vi "Calibrate pump waveplate.vi"(0 "VISA Refnum in":refnum<visa-resource-name>, 1 "Trigger rate \nat maximum":dbl, 2 "Mode":enum16{"Constant power", "Constant time"}(ring), 3 "Trigger rate warnings?":bool, 5 "Target trial \nlength (ms)":dbl, 7 "Target trigger rate":dbl, 8 "Threshold":dbl, 9 "Photon #":i32, 11 "error in (no error)":errorcluster, 13 "N":i32=5, 14 "Axis in":i32=3) -> (4 "VISA Refnum out":refnum<visa-resource-name>, 6 "WP position":dbl, 10 "WP Error":bool=TRUE, 15 "error out":errorcluster)   [LabVIEW 2013]
uses:
  <vilib>/imath/engines/lvmath2/RunTimeEngine/BuiltInFunctions/asin/NIMS_asin(C).vi
  <instcachedir>/0/NIMS_asin(C)_73B68F6B04904A8785972686F67E90FD.lvgen/NIMS_asin(C)_73B68F6B04904A8785972686F67E90FD_001.vi
  <vilib>/imath/engines/lvmath2/RunTimeEngine/NodeEndStatement/NIMS_NodeEndStatement_Output.vi
  <instcachedir>/0/NIMS_NodeEndStatement_Output_53EC0D466D134D7ABD903AC30B43404B.lvgen/NIMS_NodeEndStatement_Output_53EC0D466D134D7ABD903AC30B43404B_010.vi
  <instcachedir>/0/NIMS_NodeEndStatement_Output_53EC0D466D134D7ABD903AC30B43404B.lvgen/NIMS_NodeEndStatement_Output_53EC0D466D134D7ABD903AC30B43404B_001.vi
  <vilib>/imath/engines/lvmath2/RunTimeEngine/BuiltInFunctions/abs/NIMS_abs(signed).vi
  <instcachedir>/0/NIMS_abs(signed)_C4FCB8E6058B49B797C7C8D53CA5F6EC.lvgen/NIMS_abs(signed)_C4FCB8E6058B49B797C7C8D53CA5F6EC_000.vi
  <vilib>/imath/engines/lvmath2/RunTimeEngine/ErrorHandling/NIMS_Finalize Error.vi
  <instcachedir>/0/NIMS_NodeEndStatement_Output_53EC0D466D134D7ABD903AC30B43404B.lvgen/NIMS_NodeEndStatement_Output_53EC0D466D134D7ABD903AC30B43404B_009.vi
  <instcachedir>/0/NIMS_abs(signed)_C4FCB8E6058B49B797C7C8D53CA5F6EC.lvgen/NIMS_abs(signed)_C4FCB8E6058B49B797C7C8D53CA5F6EC_002.vi
panel:
  out "t_ratio":dbl
  out "Time":dbl
  out "Calculated trial length":dbl
  out "theta1":dbl
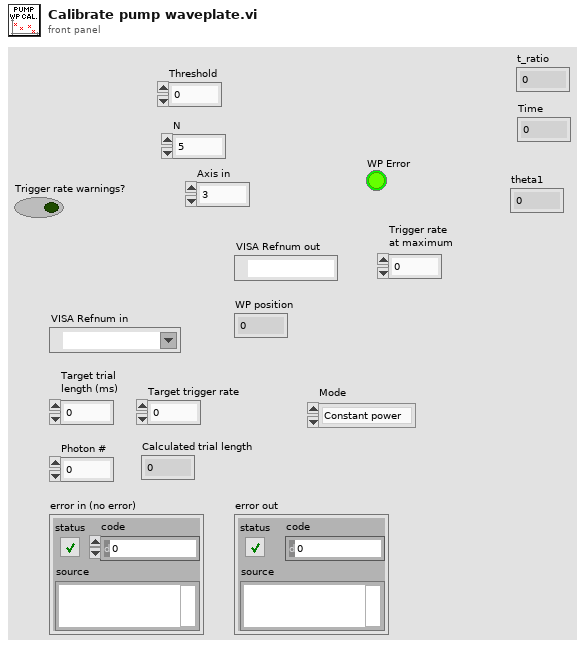
[diagram p1: front panel]
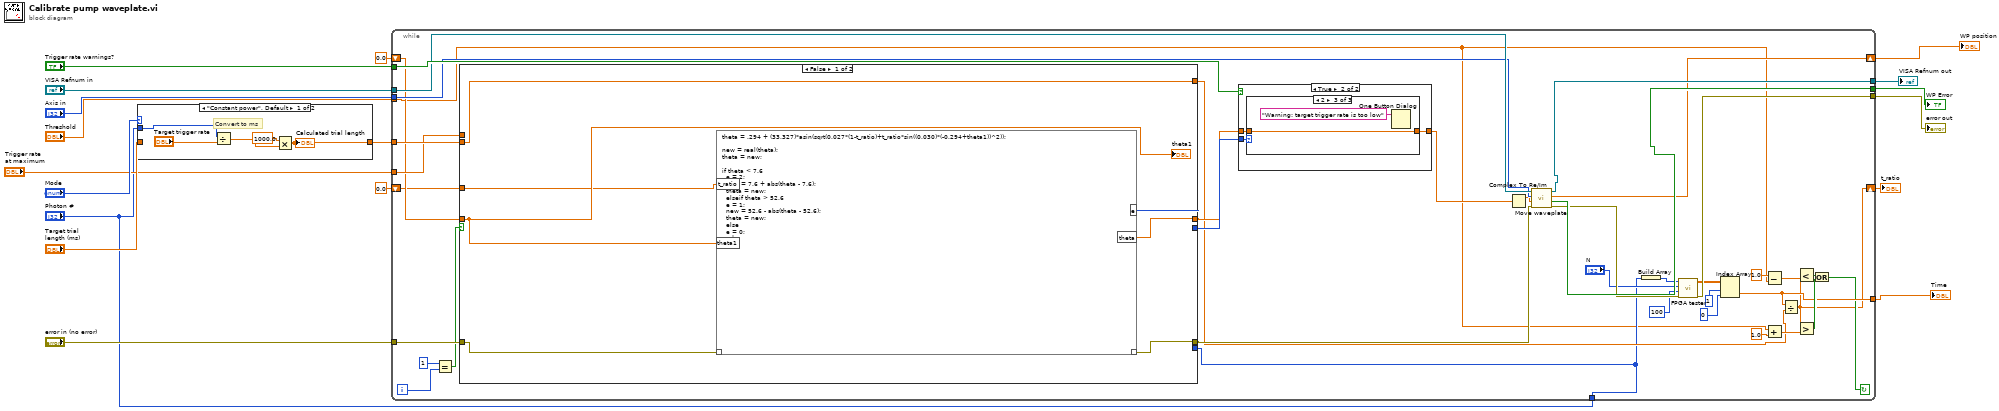
[diagram p0: block diagram]
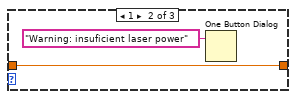
[diagram p4: hidden frame]
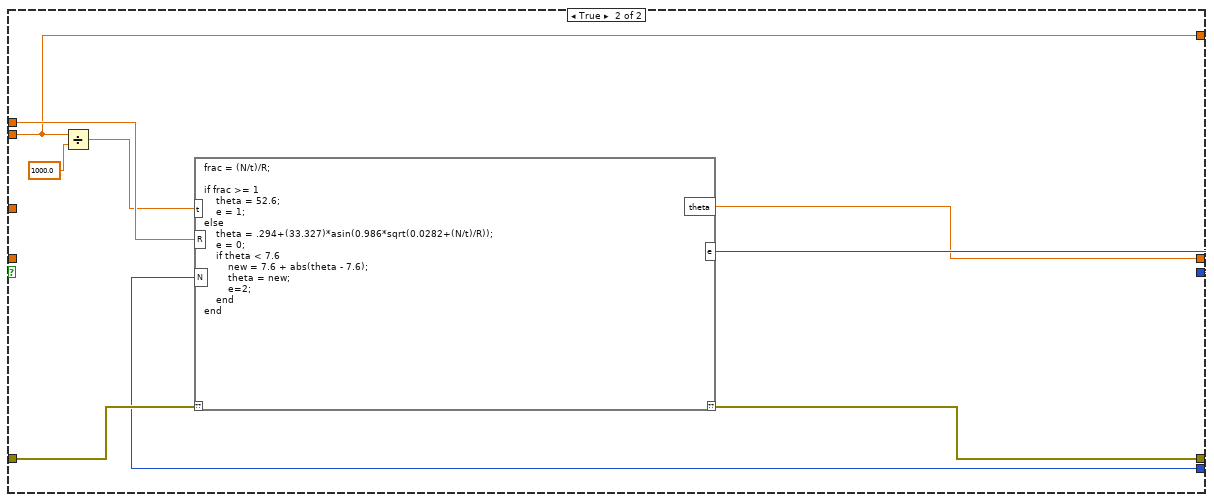
[diagram p5: hidden frame]
diagram:
  n1 = case shown="\"Constant power\", Default" "Mode" {
    tunnel: [w19 w24] -> w12
    tunnel: "Target trial \nlength (ms)" -> [_ w24]
    tunnel: "Photon #" -> [w23 _]
    frame "Constant power", Default {
      # "Convert to ms"
      n2 = Divide(x=w23, y="Target trigger rate") -> (x/y=w21:dbl)
      n3 = Multiply(x=1000.0, y=w21) -> (x*y=w19:dbl)
      "Calculated trial length" <- w19
    }
    frame "Constant time" {
    }
  }
  n4 = while {
    tunnel: "error in (no error)" -> [w63]
    tunnel: "Trigger rate warnings?" -> [w62]
    tunnel: [w61] -> w16
    tunnel: [w60] -> w15
    tunnel: [w45] -> w13
    tunnel: w12 -> [w59]
    tunnel: "Threshold" -> [w25]
    tunnel: "VISA Refnum in" -> [w49]
    tunnel: "Axis in" -> [w48]
    tunnel: "Trigger rate \nat maximum" -> [w58]
    tunnel: "Photon #" -> [w26]
    shift-right: [w50] -> w14
    shift-left: 0.0 ("Current position (units)") -> [w39]
    shift-right: [w29] -> w1
    shift-left: 0.0 -> [w28]
    tunnel: [w32] -> w4
    i -> [w53]
    stop <- w30 continue-if-true
    n5 = Equal?(x=1, y=w53) -> (x = y?=w52:bool)
    n6 = case shown="False" w52 {
      tunnel: w58 -> [_ w215]
      tunnel: [w76 w209] -> w56
      tunnel: [w79 w214] -> w57
      tunnel: w59 -> [w74 w207]
      tunnel: w63 -> [w78 w213]
      tunnel: [w77 w212] -> w51
      tunnel: w39 -> [w75 _]
      tunnel: [w74 w207] -> w31
      tunnel: w28 -> [w73 _]
      tunnel: w26 -> [_ w208]
      frame False {
        n7 = mathscript code="theta = .294 + (33.327)*asin(sqrt(0.027*(1-t_ratio)+t_ratio*sin((0.030)*(-0.294+theta1))^2));\n\nnew = real(theta);\ntheta = new;\n\nif theta < 7.6\n  e = 2;\n  new = 7.6 + abs(theta - 7.6);\n  theta = new;\n  elseif theta > 52.6\n  e = 1;\n  new = 52.6 - abs(theta - 52.6);\n  theta = new;\n  else\n  e = 0;\nend"("??"=w78, "t_ratio"=w73, "theta1"=w75) -> ("??"=w77:errorcluster, "e"=w79:i32, "theta"=w76:dbl)
        "theta1" <- w75
      }
      frame True {
        n8 = Divide(x=w207, y=1000.0) -> (x/y=w210:dbl)
        n9 = mathscript code="frac = (N/t)/R;\n\nif frac >= 1\n    theta = 52.6;\n    e = 1;\nelse\n    theta = .294+(33.327)*asin(0.986*sqrt(0.0282+(N/t)/R));\n    e = 0;\n    if theta < 7.6\n        new = 7.6 + abs(theta - 7.6);\n        theta = new;\n        e=2;\n    end\nend"("??"=w213, "t"=w210, "R"=w215, "N"=w208) -> ("??"=w212:errorcluster, "e"=w214:i32, "theta"=w209:cdb)
      }
    }
    n10 = case shown="True" w62 {
      tunnel: [w64 w67] -> w55
      tunnel: w56 -> [w64 w66]
      tunnel: w57 -> [_ w65]
      frame False {
      }
      frame True {
        n11 = case shown="2" w65 {
          tunnel: w66 -> [w68 w69 w71]
          tunnel: [w68 w69 w71] -> w67
          frame 0, Default {
          }
          frame 1 {
            n12 = One Button Dialog(message="Warning: insuficient laser power") -> ()  [unwired: 1 in, 1 out]
          }
          frame 2 {
            n13 = One Button Dialog(message="Warning: target trigger rate is too low") -> ()  [unwired: 1 in, 1 out]
          }
        }
      }
    }
    n14 = Complex To Re/Im(x + iy=w55) -> (x=w47:dbl)  [unwired: 1 out]
    n15 = call "Move waveplate.vi"("error in (no error)"=w51, "Angle"=w47, "Axis in"=w48, "VISA Refnum in"=w49) -> ("error out"=w46:errorcluster, "WP Error"=w60:bool, "Current position (units)"=w50:dbl, "VISA Refnum out"=w61:refnum<visa-resource-name>)  [unwired: 4 in]
    n16 = Build Array(w26) -> (w44:i32[])
    n17 = call "FPGA tester.vi"("error in"=w46, "Delay"=u32 100, "Repetitions"="N", "Levels"=w44) -> ("error out"=w45:errorcluster, "Results"=w41:dbl[][])  [unwired: 2 in]
    n18 = Index Array(array=w41, index (row)=1, index (col)=0 ("disabled index (col)")) -> (element=w32:dbl)
    n19 = Subtract(x=1.0 ("y"), y=w25) -> (x-y=w36:dbl)
    n20 = Add(x=w25, y=1.0) -> (x+y=w34:dbl)
    n21 = Divide(x=w32, y=w31) -> (x/y=w29:dbl)
    n22 = Less?(x=w29, y=w36) -> (x < y?=w38:bool)
    n23 = Greater?(x=w29, y=w34) -> (0:w37:bool)
    n24 = Or(x=w38, y=w37) -> (x .or. y?=w30:bool)
  }
  "WP position" <- w14
  "error out" <- w13
  "VISA Refnum out" <- w16
  "WP Error" <- w15
  "Time" <- w4
  "t_ratio" <- w1
